vi "Win3Bands.vi"() -> ()   [LabVIEW 2015]
panel:
  out "cout":string
  in  "Boule 3":u32(colorbox)
  in  "Boule 2":u32(colorbox)
  in  "Boule1":u32(colorbox)
  out "error out":errorcluster
  in  "Boule Blanche":u32=13172680 format="%.0x"
  in  "Boule  Jaune":u32=16776960 format="%.0x"
  in  "Boule Rouge":u32=16711680 format="%.0x"
  out "?":u32(colorbox)
  out "?":u32(colorbox)
  out "?":u32(colorbox)
  out "Affichage \nScoreSheet":string
  out "image":u8[](array[numeric])
  in  "path to PNG file":path
  out "new picture":picture
  out "Pixmap.bin":u32[](array[numeric])
  # "Veuillez inserer votre choix de couleurs pour le tracŽ du Plot Matlab en fonction de la boule"
  # "Couleurs des Boules"
  # "Choix des couleurs\n           du Plot"
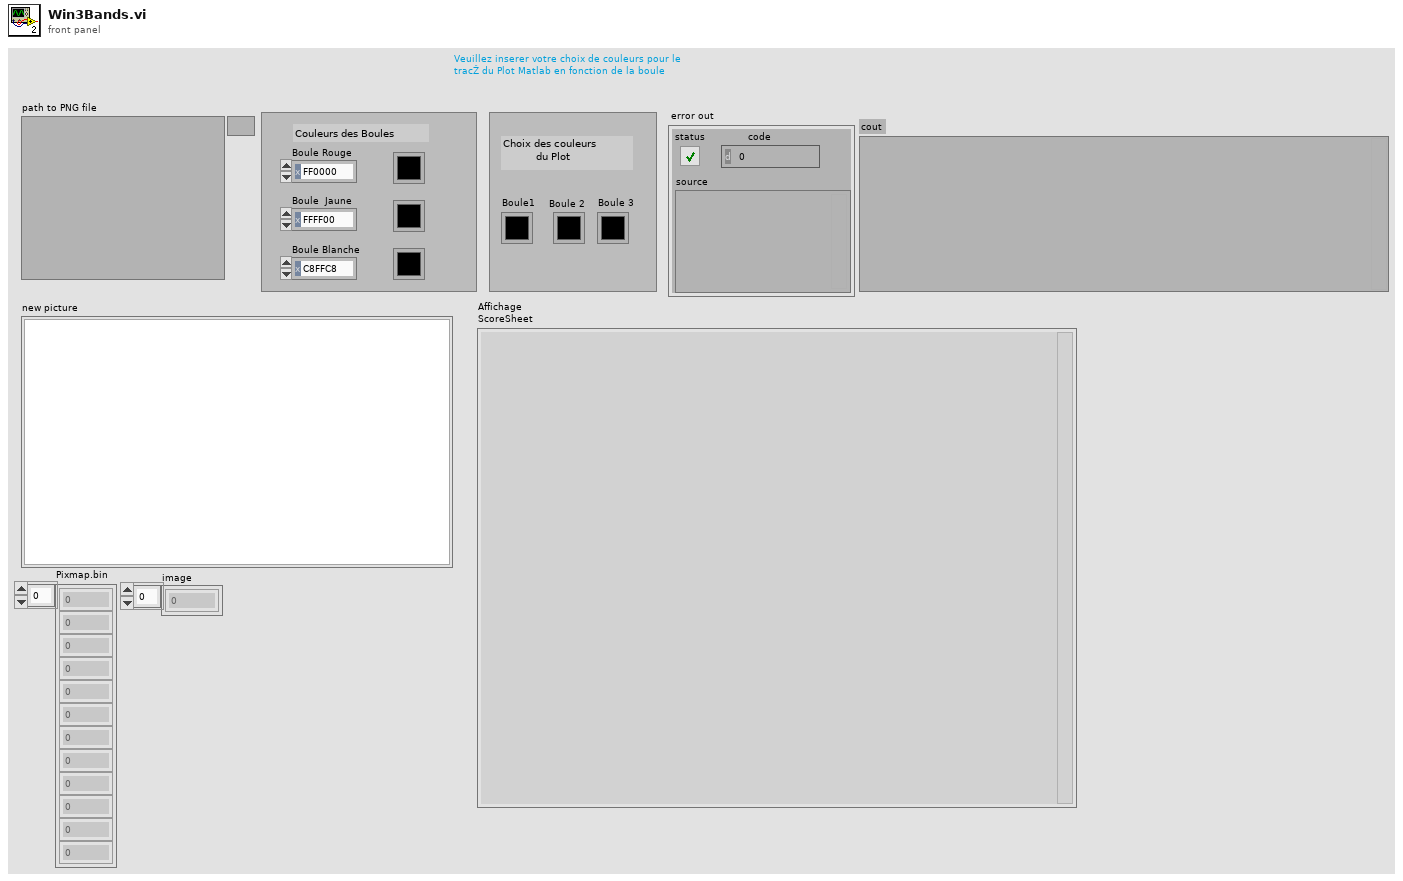
[diagram p1: front panel]
types:
  T1 = enum16{"big-endian, network order", "native, host order", "little-endian"}
  T2 = typedef "imagedata.ctl" = cluster{"image type":i32, "image depth":i32, "image":u8[], "mask":u8[], "colors":u32[], "Rectangle":cluster{"left":i16, "top":i16, "right":i16, "bottom":i16}}
  T3 = cluster{"status":bool, "code":i32, "standard error":string}
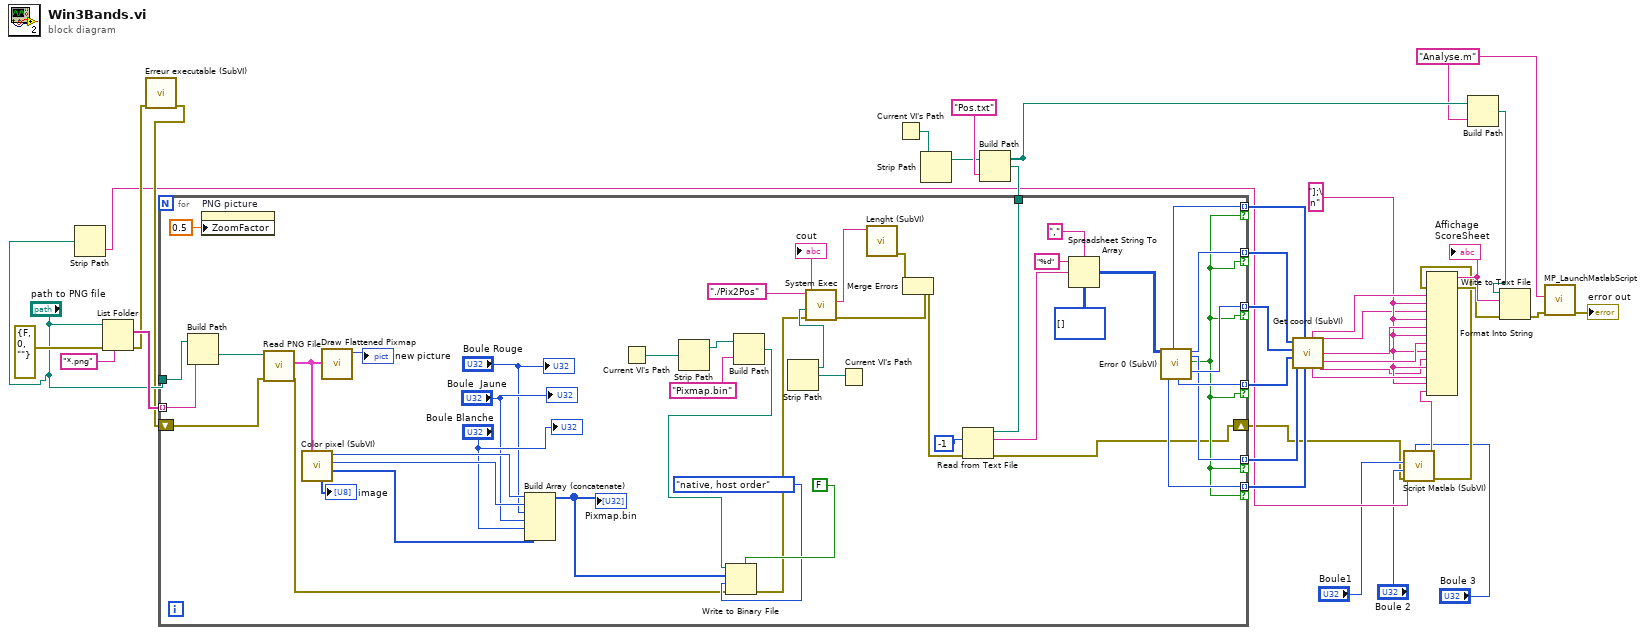
[diagram p0: block diagram]
diagram:
  w23 = "Analyse.m" ("name or relative path")
  w21 = "];\n"
  n1 = Strip Path(path="path to PNG file") -> (name=w5:string)  [unwired: 1 out]
  n2 = List Folder(path="path to PNG file", pattern="*.png", error in=errorcluster {"status"=FALSE, "code"=0, "source"=""} ("error constant")) -> (filenames=w34:string[], error out=w10:errorcluster)  [unwired: 1 in, 2 out]
  n3 = call "Erreur executable (SubVI).vi"("error in (no error)"=w10) -> ("error out"=w8:errorcluster)  [unwired: 10 in]
  n4 = Current VI's Path() -> (path=w32:path)
  n5 = Strip Path(path=w32) -> (stripped path=w25:path)  [unwired: 1 out]
  n6 = Build Path(base path=w25, name or relative path="Pos.txt") -> (appended path=w31:path)
  n7 = for {
    tunnel: "path to PNG file" -> [w69]
    tunnel: w34 -> [w68] mode=indexing
    tunnel: w31 -> [w55]
    tunnel: [w44] -> w18 mode=indexing if=w38
    tunnel: [w43] -> w17 mode=indexing if=w38
    tunnel: [w42] -> w16 mode=indexing if=w38
    tunnel: [w41] -> w15 mode=indexing if=w38
    tunnel: [w40] -> w14 mode=indexing if=w38
    tunnel: [w39] -> w13 mode=indexing if=w38
    shift-right: [w37] -> w1
    shift-left: w8 -> [w46]
    n8 = Build Path(base path=w69, name or relative path=w68) -> (appended path=w67:path)
    n9 = property on="PNG picture" class="Pict"("ZoomFactor"=sgl 0.5 ("Zoom Factor")) -> ()  [unwired: 2 in, 2 out]
    n10 = call <vilib>:"Read PNG File.vi"("error in (no error)"=w46, "path to PNG file"=w67) -> ("error out"=w65:errorcluster, "image data"=w78:T2)  [unwired: 7 in, 1 out]
    n11 = call "Color pixel (SubVI).vi"("image data"=w78) -> ("Array"=w63:u32[], "bottom"=w75:i16, "right"=w76:i16, "image"=→"image":u8[])  [unwired: 7 in]
    n12 = call <vilib>:"Draw Flattened Pixmap.vi"("image data"=w78) -> ("new picture"=→"new picture":picture)  [unwired: 8 in]
    n13 = Build Array (concatenate)(w76, w75, "Boule Rouge", "Boule  Jaune", "Boule Blanche", w63) -> (w77:u32[])
    "Pixmap.bin" <- w77
    n14 = Current VI's Path() -> (path=w73:path)
    n15 = Strip Path(path=w73) -> (stripped path=w72:path)  [unwired: 1 out]
    n16 = Build Path(base path=w72, name or relative path="Pixmap.bin") -> (appended path=w70:path)
    n17 = Write to Binary File(file (use dialog)=w70, data=w77, error in=w65, 5:FALSE, 9:T1."native, host order" ("byte order (0:big-endian, network order)")) -> (error out=w64:errorcluster)  [unwired: 1 in, 2 out]
    n18 = Current VI's Path() -> (path=w74:path)
    n19 = Strip Path(path=w74) -> (stripped path=w66:path)  [unwired: 1 out]
    n20 = call <vilib>:"System Exec.vi"("error in (no error)"=w64, "working directory"=w66, "command line"="./Pix2Pos") -> ("error out"=w54:errorcluster, "standard error"=w51:string, "standard output"=→"cout":string)  [unwired: 5 in, 1 out]
    n21 = call "Lenght (SubVI).vi"("standard error"=w51) -> ("error out"=w52:T3)  [unwired: 10 in]
    n22 = Merge Errors(w52, w54) -> (w56:errorcluster)
    n23 = Read from Text File(file (use dialog)=w55, count=-1, error in=w56) -> (text=w59:string, error out=w37:errorcluster)  [unwired: 1 in, 2 out]
    n24 = Spreadsheet String To Array(delimiter (Tab)=",", format string="%d", spreadsheet string=w59, array type (2D Dbl)=i32[][] []) -> (array=w50:i32[][])
    n25 = call "Error 0 (SubVI).vi"("array type (2D Dbl)"=w50) -> ("Numeric"=w39:i32, "Numeric 6"=w44:i32, "Numeric 3"=w41:i32, "Numeric 5"=w43:i32, "Numeric 2"=w40:i32, "result"=w38:bool, "Numeric 4"=w42:i32)  [unwired: 12 in]
    "?" <- "Boule Rouge"
    "?" <- "Boule  Jaune"
    "?" <- "Boule Blanche"
  }
  n26 = call "Get coord (SubVI).vi"("Array"=w13, "Array 6"=w18, "Array 2"=w14, "Array 3"=w15, "Array 4"=w16, "Array 5"=w17) -> ("String 2"=w19:string, "String 3"=w28:string, "String 4"=w29:string, "String 5"=w20:string, "String"=w27:string, "String 6"=w33:string)
  n27 = call "Script Matlab (SubVI).vi"("Color 3"="Boule 3", "error in (no error)"=w1, "Color 2"="Boule 2", "Color"="Boule1", "name"=w5) -> ("error out"=w6:errorcluster, "String"=w7:string)  [unwired: 5 in]
  n28 = Format Into String(error in=w6, w33, w21, w20, w21, w29, w21, w28, w21, w19, w21, w27, w21, w7) -> (resulting string=w26:string, error out=w11:errorcluster)  [unwired: 2 in]
  "Affichage \nScoreSheet" <- w26
  n29 = Build Path(base path=w25, name or relative path=w23) -> (appended path=w24:path)
  n30 = Write to Text File(file (use dialog)=w24, text=w26, error in=w11) -> (error out=w22:errorcluster)  [unwired: 1 in, 2 out]
  n31 = call "MP_LaunchMatlabScript.vi"("error in (no error)"=w22, "matlab script name with extension"=w23) -> ("error out"=→"error out":errorcluster)  [unwired: 5 in, 4 out]
